vi "Untitled 7.vi"() -> ()   [LabVIEW 2017]
uses:
  <vilib>/Utility/miscctls.llb/LVPositionTypeDef.ctl
  <vilib>/Utility/miscctls.llb/LVBoundsTypeDef.ctl
panel:
  in  "Cross? Button":bool
  in  "Three Cube Button":bool
  in  "Two Cube Button":bool
  in  "One Cube Button":bool
  in  "Switch Button":bool
  in  "Scale Button":bool
  in  "Right Button":bool
  in  "Center Button":bool
  in  "Left Button":bool
  out "StartPos":string
  out "Priority":string
  out "NumCubes":string
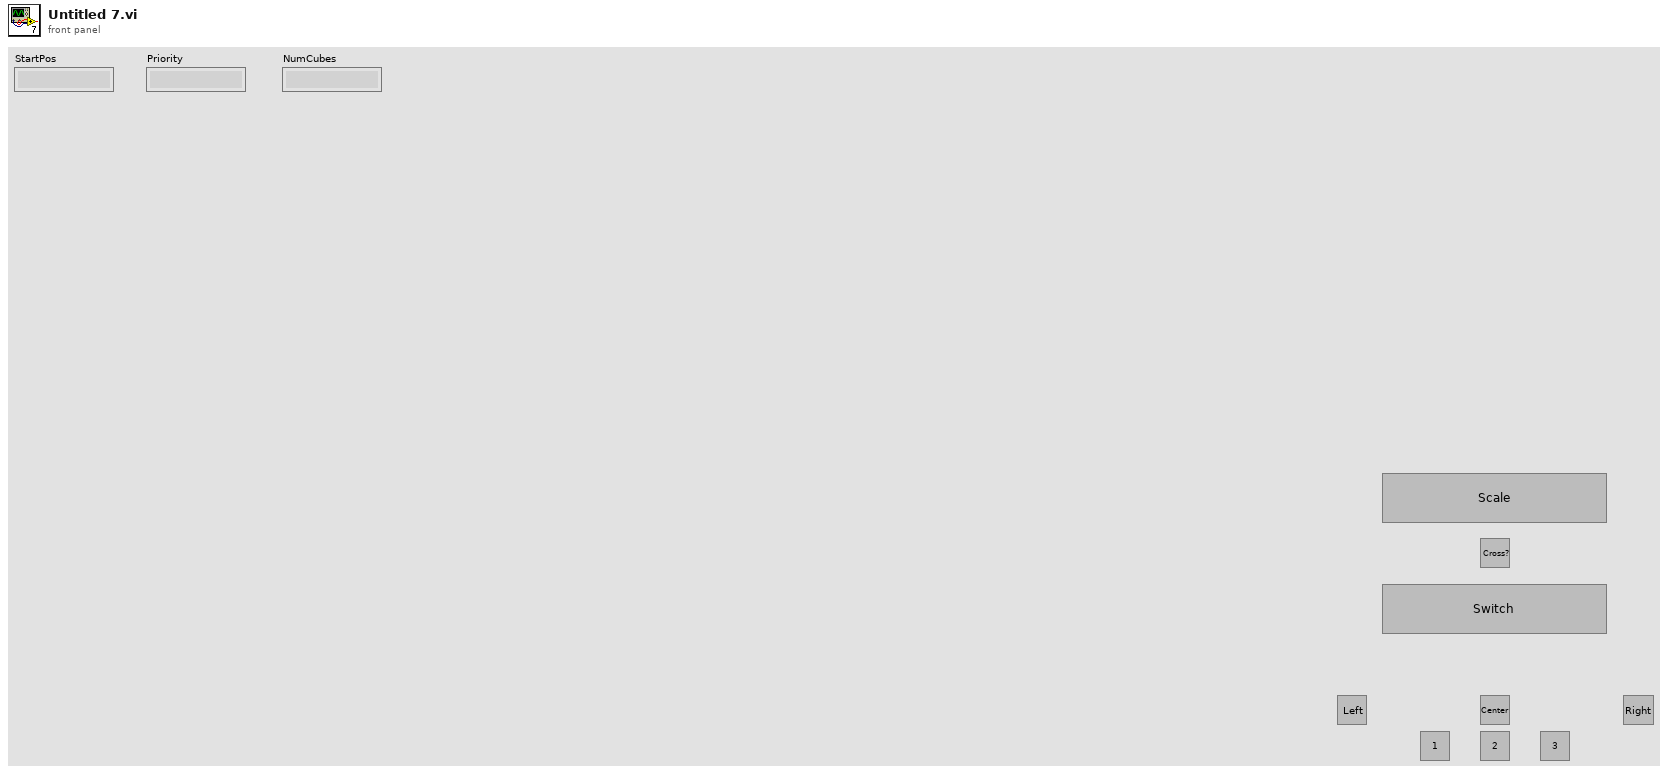
[diagram p1: front panel]
types:
  T1 = typedef "LVBoundsTypeDef.ctl" = cluster{"Width":u32, "Height":u32}
  T2 = typedef "LVPositionTypeDef.ctl" = cluster{"Left":i32, "Top":i32}
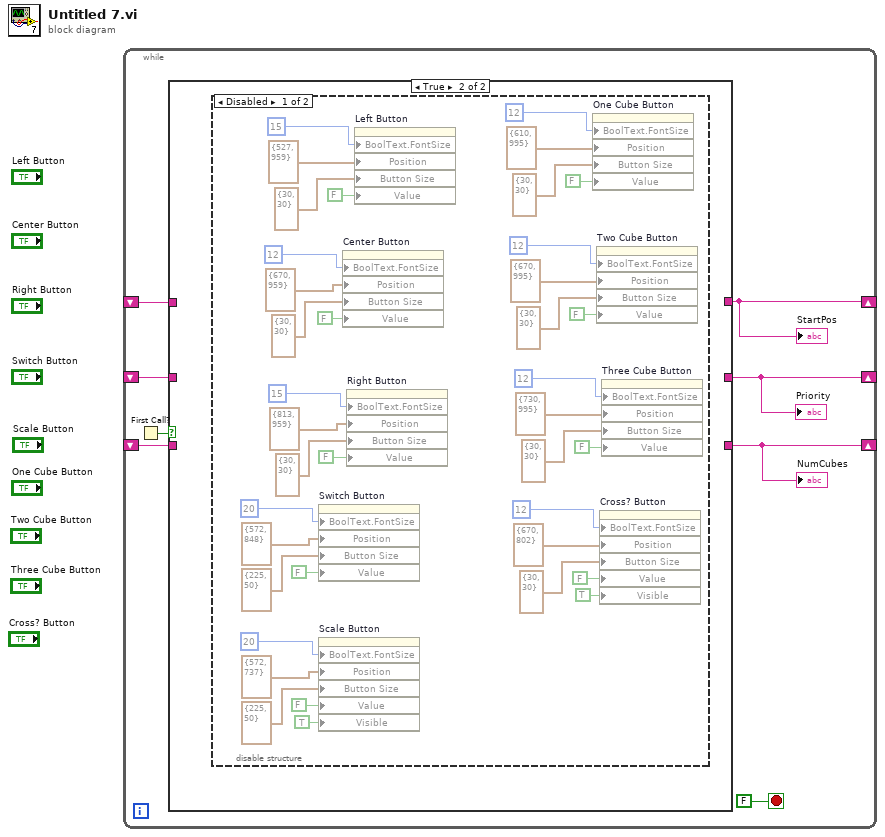
[diagram p0: block diagram]
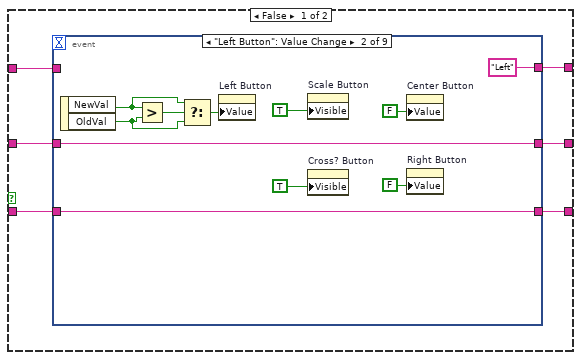
[diagram p2: hidden frame]
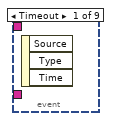
[diagram p3: hidden frame]
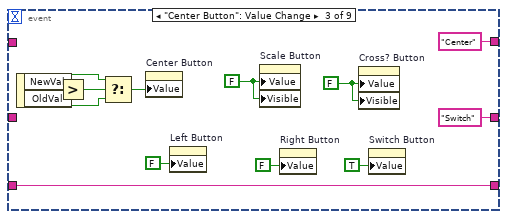
[diagram p4: hidden frame]
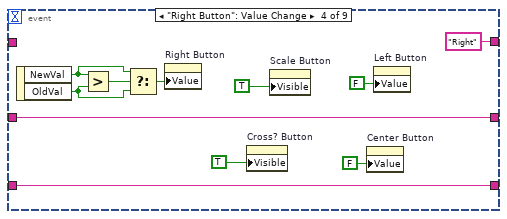
[diagram p5: hidden frame]
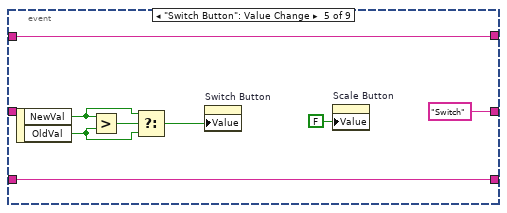
[diagram p6: hidden frame]
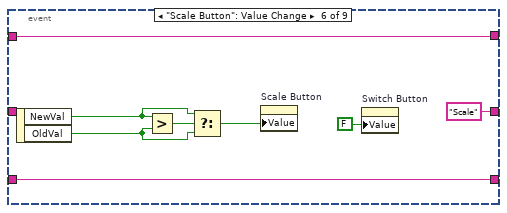
[diagram p7: hidden frame]
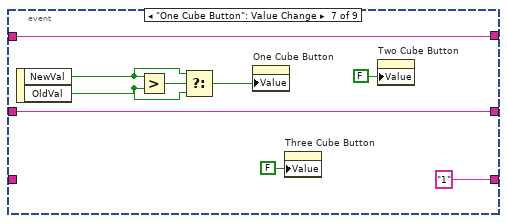
[diagram p8: hidden frame]
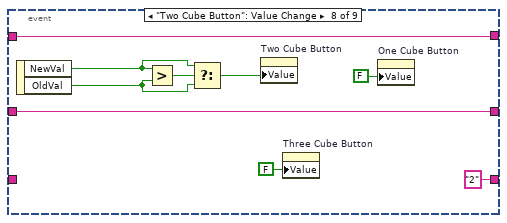
[diagram p9: hidden frame]
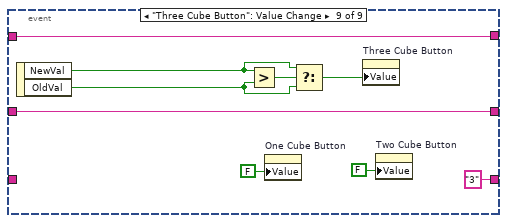
[diagram p10: hidden frame]
diagram:
  n1 = while {
    shift-right: [w5] -> _
    shift-left: _ -> [w4]
    shift-right: [w6] -> _
    shift-left: _ -> [w3]
    shift-right: [w7] -> _
    shift-left: _ -> [w2]
    stop <- FALSE stop-if-true
    n2 = First Call?() -> (First Call?: T/F=w8:bool)
    n3 = case shown="True" w8 {
      tunnel: [w14 _] -> w5
      tunnel: [w13 _] -> w6
      tunnel: [w12 _] -> w7
      tunnel: w4 -> [w11 _]
      tunnel: w3 -> [w10 _]
      tunnel: w2 -> [w9 _]
      frame False {
        n4 = event shown="[1] \"Left Button\": Value Change" {
          selector: _ -> [_ _ _ _ _ _ _ _ _]
          dyn-events: _ -> [_ _ _ _ _ _ _ _ _]
          timeout: _ -> [_ _ _ _ _ _ _ _ _]
          tunnel: [_ "Left" "Center" "Right" w50 w58 w66 w74 w84] -> w14
          tunnel: [_ w16 "Switch" w39 "Switch" "Scale" w65 w75 w83] -> w13
          tunnel: [_ w15 w27 w38 w49 w57 "1" "2" "3"] -> w12
          tunnel: w11 -> [_ _ _ _ w50 w58 w66 w74 w84]
          tunnel: w10 -> [_ w16 _ w39 _ _ w65 w75 w83]
          tunnel: w9 -> [_ w15 w27 w38 w49 w57 _ _ _]
          event Timeout {
            n5 = event-data() -> ()  [unwired: 1 in, 3 out]
          }
          event "Left Button": Value Change {
            n6 = event-data() -> ("NewVal"=w22:bool, "OldVal"=w21:bool)  [unwired: 1 in]
            n7 = Greater?(x=w22, y=w21) -> (0:w23:bool)
            n8 = Select(t=w22, s=w23, f=w21) -> (s? t:f=w20:bool)
            n9 = property on="Left Button" class="Bool (strict)"("Value"=w20) -> ()  [unwired: 2 in, 2 out]
            n10 = property on="Scale Button" class="Bool (strict)"("Visible"=TRUE ("Right Button")) -> ()  [unwired: 2 in, 2 out]
            n11 = property on="Cross? Button" class="Bool (strict)"("Visible"=TRUE ("Right Button")) -> ()  [unwired: 2 in, 2 out]
            n12 = property on="Center Button" class="Bool (strict)"("Value"=FALSE ("Center Button")) -> ()  [unwired: 2 in, 2 out]
            n13 = property on="Right Button" class="Bool (strict)"("Value"=FALSE ("Right Button")) -> ()  [unwired: 2 in, 2 out]
          }
          event "Center Button": Value Change {
            w30 = FALSE ("Right Button")
            w29 = FALSE ("Right Button")
            n14 = event-data() -> ("NewVal"=w32:bool, "OldVal"=w33:bool)  [unwired: 1 in]
            n15 = Greater?(x=w32, y=w33) -> (0:w35:bool)
            n16 = Select(t=w32, s=w35, f=w33) -> (s? t:f=w34:bool)
            n17 = property on="Center Button" class="Bool (strict)"("Value"=w34) -> ()  [unwired: 2 in, 2 out]
            n18 = property on="Left Button" class="Bool (strict)"("Value"=FALSE ("Center Button")) -> ()  [unwired: 2 in, 2 out]
            n19 = property on="Scale Button" class="Bool (strict)"("Value"=w29, "Visible"=w29) -> ()  [unwired: 2 in, 2 out]
            n20 = property on="Right Button" class="Bool (strict)"("Value"=FALSE ("Right Button")) -> ()  [unwired: 2 in, 2 out]
            n21 = property on="Cross? Button" class="Bool (strict)"("Value"=w30, "Visible"=w30) -> ()  [unwired: 2 in, 2 out]
            n22 = property on="Switch Button" class="Bool (strict)"("Value"=TRUE ("Right Button")) -> ()  [unwired: 2 in, 2 out]
          }
          event "Right Button": Value Change {
            n23 = event-data() -> ("NewVal"=w43:bool, "OldVal"=w44:bool)  [unwired: 1 in]
            n24 = Greater?(x=w43, y=w44) -> (0:w46:bool)
            n25 = Select(t=w43, s=w46, f=w44) -> (s? t:f=w45:bool)
            n26 = property on="Right Button" class="Bool (strict)"("Value"=w45) -> ()  [unwired: 2 in, 2 out]
            n27 = property on="Cross? Button" class="Bool (strict)"("Visible"=TRUE ("Right Button")) -> ()  [unwired: 2 in, 2 out]
            n28 = property on="Scale Button" class="Bool (strict)"("Visible"=TRUE ("Right Button")) -> ()  [unwired: 2 in, 2 out]
            n29 = property on="Center Button" class="Bool (strict)"("Value"=FALSE ("Right Button")) -> ()  [unwired: 2 in, 2 out]
            n30 = property on="Left Button" class="Bool (strict)"("Value"=FALSE ("Center Button")) -> ()  [unwired: 2 in, 2 out]
          }
          event "Switch Button": Value Change {
            n31 = event-data() -> ("NewVal"=w52:bool, "OldVal"=w53:bool)  [unwired: 1 in]
            n32 = Greater?(x=w52, y=w53) -> (0:w55:bool)
            n33 = Select(t=w52, s=w55, f=w53) -> (s? t:f=w54:bool)
            n34 = property on="Switch Button" class="Bool (strict)"("Value"=w54) -> ()  [unwired: 2 in, 2 out]
            n35 = property on="Scale Button" class="Bool (strict)"("Value"=FALSE ("Center Button")) -> ()  [unwired: 2 in, 2 out]
          }
          event "Scale Button": Value Change {
            n36 = event-data() -> ("NewVal"=w60:bool, "OldVal"=w61:bool)  [unwired: 1 in]
            n37 = Greater?(x=w60, y=w61) -> (0:w63:bool)
            n38 = Select(t=w60, s=w63, f=w61) -> (s? t:f=w62:bool)
            n39 = property on="Scale Button" class="Bool (strict)"("Value"=w62) -> ()  [unwired: 2 in, 2 out]
            n40 = property on="Switch Button" class="Bool (strict)"("Value"=FALSE ("Center Button")) -> ()  [unwired: 2 in, 2 out]
          }
          event "One Cube Button": Value Change {
            n41 = event-data() -> ("NewVal"=w69:bool, "OldVal"=w70:bool)  [unwired: 1 in]
            n42 = Greater?(x=w69, y=w70) -> (0:w72:bool)
            n43 = Select(t=w69, s=w72, f=w70) -> (s? t:f=w71:bool)
            n44 = property on="One Cube Button" class="Bool (strict)"("Value"=w71) -> ()  [unwired: 2 in, 2 out]
            n45 = property on="Three Cube Button" class="Bool (strict)"("Value"=FALSE ("Center Button")) -> ()  [unwired: 2 in, 2 out]
            n46 = property on="Two Cube Button" class="Bool (strict)"("Value"=FALSE ("Center Button")) -> ()  [unwired: 2 in, 2 out]
          }
          event "Two Cube Button": Value Change {
            n47 = event-data() -> ("NewVal"=w78:bool, "OldVal"=w79:bool)  [unwired: 1 in]
            n48 = Greater?(x=w78, y=w79) -> (0:w81:bool)
            n49 = Select(t=w78, s=w81, f=w79) -> (s? t:f=w80:bool)
            n50 = property on="Two Cube Button" class="Bool (strict)"("Value"=w80) -> ()  [unwired: 2 in, 2 out]
            n51 = property on="Three Cube Button" class="Bool (strict)"("Value"=FALSE ("Center Button")) -> ()  [unwired: 2 in, 2 out]
            n52 = property on="One Cube Button" class="Bool (strict)"("Value"=FALSE ("Center Button")) -> ()  [unwired: 2 in, 2 out]
          }
          event "Three Cube Button": Value Change {
            n53 = event-data() -> ("NewVal"=w87:bool, "OldVal"=w88:bool)  [unwired: 1 in]
            n54 = Greater?(x=w87, y=w88) -> (0:w90:bool)
            n55 = property on="One Cube Button" class="Bool (strict)"("Value"=FALSE ("Center Button")) -> ()  [unwired: 2 in, 2 out]
            n56 = Select(t=w87, s=w90, f=w88) -> (s? t:f=w89:bool)
            n57 = property on="Three Cube Button" class="Bool (strict)"("Value"=w89) -> ()  [unwired: 2 in, 2 out]
            n58 = property on="Two Cube Button" class="Bool (strict)"("Value"=FALSE ("Center Button")) -> ()  [unwired: 2 in, 2 out]
          }
        }
      }
      frame True {
        n59 = disable-structure shown="Disabled" {
          frame Disabled {
            n60 = property on="Switch Button" class="Bool (strict)"("BoolText.FontSize"=u32 20 ("Caption.Font:Size"), "Position"=T2 {"Left"=572, "Top"=848}, "Button Size"=T1 {"Width"=225, "Height"=50}, "Value"=FALSE) -> ()  [unwired: 2 in, 2 out]
            n61 = property on="Scale Button" class="Bool (strict)"("BoolText.FontSize"=u32 20 ("Caption.Font:Size"), "Position"=T2 {"Left"=572, "Top"=737}, "Button Size"=T1 {"Width"=225, "Height"=50}, "Value"=FALSE, "Visible"=TRUE) -> ()  [unwired: 2 in, 2 out]
            n62 = property on="Center Button" class="Bool (strict)"("BoolText.FontSize"=u32 12 ("Caption.Font:Size"), "Position"=T2 {"Left"=670, "Top"=959}, "Button Size"=T1 {"Width"=30, "Height"=30}, "Value"=FALSE) -> ()  [unwired: 2 in, 2 out]
            n63 = property on="Right Button" class="Bool (strict)"("BoolText.FontSize"=u32 15 ("Caption.Font:Size"), "Position"=T2 {"Left"=813, "Top"=959}, "Button Size"=T1 {"Width"=30, "Height"=30}, "Value"=FALSE) -> ()  [unwired: 2 in, 2 out]
            n64 = property on="Left Button" class="Bool (strict)"("BoolText.FontSize"=u32 15 ("Caption.Font:Size"), "Position"=T2 {"Left"=527, "Top"=959}, "Button Size"=T1 {"Width"=30, "Height"=30}, "Value"=FALSE) -> ()  [unwired: 2 in, 2 out]
            n65 = property on="One Cube Button" class="Bool (strict)"("BoolText.FontSize"=u32 12 ("Caption.Font:Size"), "Position"=T2 {"Left"=610, "Top"=995}, "Button Size"=T1 {"Width"=30, "Height"=30}, "Value"=FALSE) -> ()  [unwired: 2 in, 2 out]
            n66 = property on="Two Cube Button" class="Bool (strict)"("BoolText.FontSize"=u32 12 ("Caption.Font:Size"), "Position"=T2 {"Left"=670, "Top"=995}, "Button Size"=T1 {"Width"=30, "Height"=30}, "Value"=FALSE) -> ()  [unwired: 2 in, 2 out]
            n67 = property on="Cross? Button" class="Bool (strict)"("BoolText.FontSize"=u32 12 ("Caption.Font:Size"), "Position"=T2 {"Left"=670, "Top"=802}, "Button Size"=T1 {"Width"=30, "Height"=30}, "Value"=FALSE, "Visible"=TRUE) -> ()  [unwired: 2 in, 2 out]
            n68 = property on="Three Cube Button" class="Bool (strict)"("BoolText.FontSize"=u32 12 ("Caption.Font:Size"), "Position"=T2 {"Left"=730, "Top"=995}, "Button Size"=T1 {"Width"=30, "Height"=30}, "Value"=FALSE) -> ()  [unwired: 2 in, 2 out]
          }
          frame Enabled {
          }
        }
      }
    }
    "StartPos" <- w5
    "Priority" <- w6
    "NumCubes" <- w7
  }
